vi "Robot Global Data.vi"() -> ()   [LabVIEW 2018]
doc: "This global VI can contain as many global variables as you need. Place a control on the panel, give it a good name. To read or write to it from a VI, drag the icon to the diagram of that VI. You can also drag from the project. Click on the node to change which global you access. You shouldn't have multiple locations writing to a global or it will cause a race-condition."
uses:
  <vilib>/Rock Robotics/WPI/Camera/WPI_CameraImageSize.ctl
  <vilib>/Rock Robotics/WPI/DriverStation/WPI_DriverStationRobotMode2.ctl
panel:
  in  "COLUNA":dbl
  in  "LINHA":dbl
  in  "Array":T1(array[ring])
  in  "ESQ/DIR":dbl
  in  "ANGULO ENTREGA":dbl=1100.0
  in  "ALTURA ENTREGA":dbl=1100.0
  out "ALTURA MEDIA":bool=TRUE
  out "PEGOU BOLA":bool=TRUE
  in  "SAÍDA GARRA FRENTE":dbl
  out "GARRA FRENTE RECUA":bool=TRUE
  out "GARRA FRENTE AVANÇA":bool=TRUE
  in  "PROCESSO":bool
  in  "POSI敲O ATUAL GAR":dbl=5.0
  out "CHEGOU GARRA":bool=TRUE
  out "CHEGOU ELEVADOR":bool=TRUE
  out "pegou":bool
  out "DISCO":bool
  out "BOLA":bool
  out "SOLTA":bool
  out "PEGA":bool
  out "ESQUERDA":bool
  out "DIREITA":bool
  out "SUPERIOR":bool
  out "MEDIO":bool
  out "RECUA PISTÃO":bool
  out "AVANÇA PISTÃO":bool
  in  "SAÍDA PID DIREITO":dbl
  in  "SAÍDA PID ESQUERDO":dbl
  in  "VALOR GIRO GARRA":dbl
  in  "POSI敲O ELEVADOR":dbl=1103.0
  in  "OFFSET ELEVADOR":dbl=1103.0
  in  "MOTOR BOLA":dbl
  in  "GAIN":T2
  out "VELOCIDADE ZERO":bool
  in  "POSI敲O DE PEGAR":dbl
  in  "VELOCIDADE FREZOS":dbl
  in  "VELOCIDADE ELEVADOR":dbl
  in  "VELOCIDADE GIRA GARRA":dbl
  in  "VELOCIDADE GARRA FRENTE":dbl=-0.6
  in  "Posição garra frente":dbl=-0.25
  in  "MANCHE2":dbl
  in  "MANCHE1":dbl
  in  "POSI敲O GAR.":dbl=5.0
  in  "POSI敲O":dbl=1100.0
  in  "Robot Mode":T3=enum."Teleop Enabled"
  in  "image size":T4=enum."320x240"
  in  "Enable Vision":bool
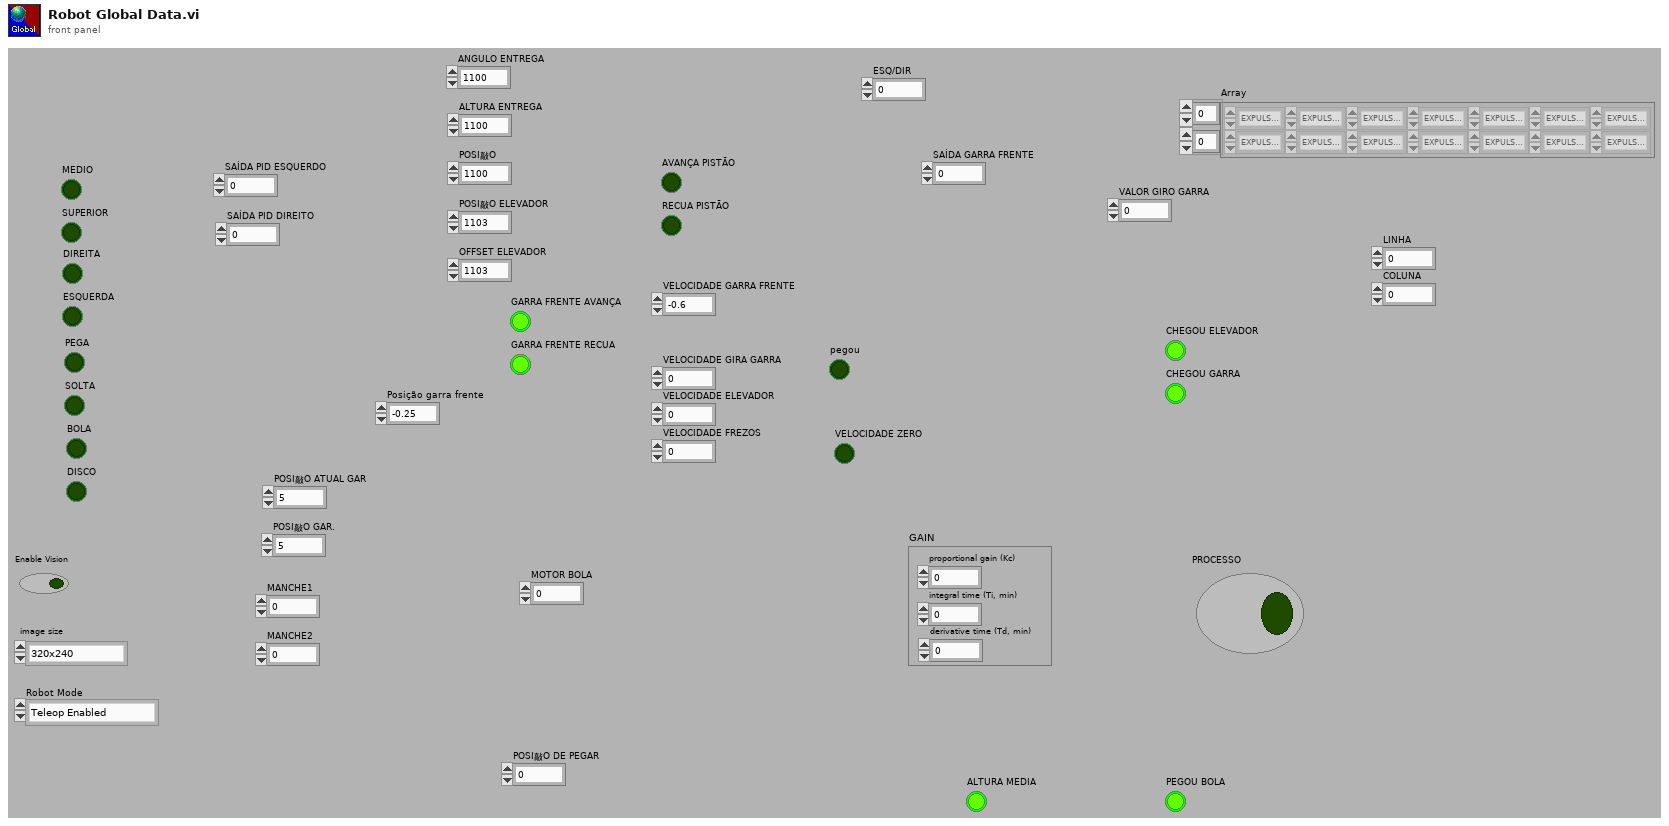
[diagram p1: front panel]
types:
  T1 = enum16{"EXPULSA DISCO", "EXPULSA BOLA", "POSI敲O ENTREGA", "PEGAR BOLA", "POSI敲O NEUTRA", "DESCE ELEVADOR", "TERMINA SEQUENCIA"}[][]
  T2 = cluster{"proportional gain (Kc)":dbl, "integral time (Ti, min)":dbl, "derivative time (Td, min)":dbl}
  T3 = typedef "WPI_DriverStationRobotMode2.ctl" = enum16{"Autonomous Disabled", "Autonomous Enabled", "Teleop Disabled", "Teleop Enabled", "Disconnected", "Finish", "Test Disabled", "Test Enabled", "Emergency Stopped"}
  T4 = typedef "WPI_CameraImageSize.ctl" = enum16{"640x480", "320x240", "160x120", "Custom"}
diagram:
